vi "DeviceNet Write Data.vi"() -> ()   [LabVIEW 2010]
uses:
  <vilib>/nidnet/Nidnet.llb/DnetIntfConfig.ctl
panel:
  in  "DeviceNet Interface Configuration":T1 {"IntfMacId" max=63 step=1}
  out "Error out":errorcluster {"code" format="%.0x"}
  in  "Error in":errorcluster {"code" format="%.0x"}
  in  "IntfName":T2(ring)
  in  "ByteOffset":u16
  in  "String Input":string
  in  "DBL/SGL in":dbl format="%.2f"
  in  "8[TF] in":bool[](array[boolean])
  in  "I32/I16/I8 in":i32
  in  "U32/U16/U8 in":u32
  in  "Dnet Input Type":T3(ring)
  in  "DnetData in":u8[](array[numeric])
  # "DeviceNet Write Data"
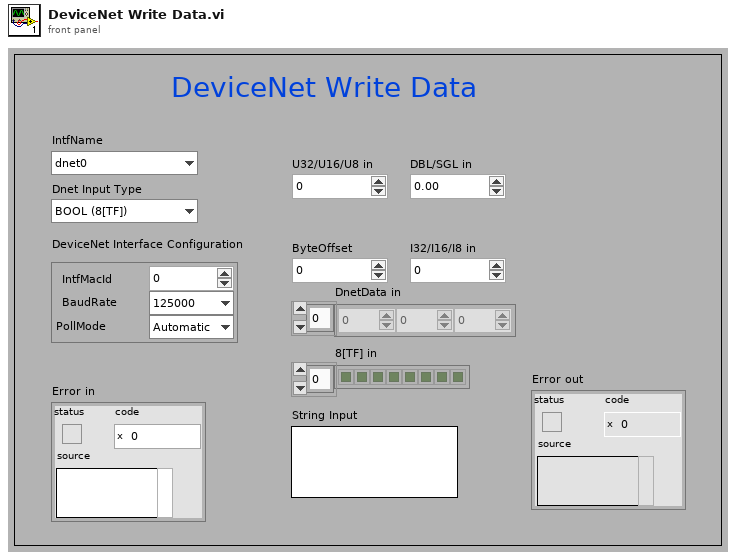
[diagram p1: front panel]
types:
  T1 = typedef "DnetIntfConfig.ctl" = cluster{"IntfMacId":u32, "BaudRate":enum32{"125000", "250000", "500000"}, "PollMode":enum32{"Automatic", "Scanned", "Individual"}}
  T2 = enum16{"dnet0", "dnet1", "dnet2", "dnet3", "dnet4", "dnet5", "dnet6", "dnet7", "dnet8", "dnet9", "dnet10", "dnet11", "dnet12", "dnet13", "dnet14", "dnet15", "dnet16", "dnet17", "dnet18", "dnet19", "dnet20", "dnet21", "dnet22", "dnet23", "dnet24", "dnet25", "dnet26", "dnet27", "dnet28", "dnet29", "dnet30", "dnet31"}
  T3 = enum16{"BOOL (8[TF])", "SINT (I8)", "INT (I16)", "DINT (I32)", "USINT (U8)", "UINT (U16)", "UDINT (U32)", "REAL (SGL)", "LREAL (DBL)", "SHORT_STRING (abc)", "STRING (abc)"}
  T4 = typedef "xobjhandle.ctl" = u32
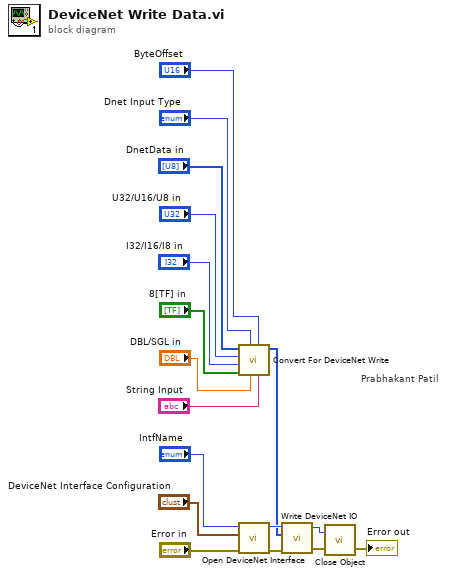
[diagram p0: block diagram]
diagram:
  # "Prabhakant Patil"
  n1 = call <vilib>:"Convert For DeviceNet Write.vi"("abc in"="String Input", "ByteOffset"="ByteOffset", "DBL/SGL in"="DBL/SGL in", "DnetType"="Dnet Input Type", "8[TF] in"="8[TF] in", "I32/I16/I8 in"="I32/I16/I8 in", "U32/U16/U8 in"="U32/U16/U8 in", "DnetData in"="DnetData in") -> ("DnetData out"=w16:u8[])  [unwired: 3 in]
  n2 = call <vilib>:"Open DeviceNet Interface.vi"("Error in"="Error in", "DeviceNet Interface Configuration"="DeviceNet Interface Configuration", "IntfName"="IntfName") -> ("Error out"=w14:errorcluster, "ObjHandle out"=w17:T4)  [unwired: 3 in]
  n3 = call <vilib>:"Write DeviceNet IO.vi"("ObjHandle in"=w17, "Data"=w16, "Error in"=w14) -> ("ObjHandle out"=w13:T4, "Error out"=w12:errorcluster)  [unwired: 3 in]
  n4 = call <vilib>:"Close Object.vi"("Error in"=w12, "ObjHandle in"=w13) -> ("Error out"=→"Error out":errorcluster)  [unwired: 1 in]
